vi "FilePath.vi"() -> (3 "添加的路径":path)   [LabVIEW 2018]
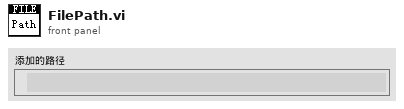
[diagram p1: front panel]
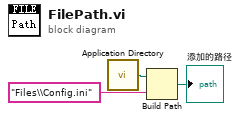
[diagram p0: block diagram]
diagram:
  n1 = call <vilib>:"Application Directory.vi"() -> ("Application Directory"=w3:path)
  n2 = Build Path(base path=w3, name or relative path="Files\\Config.ini" ("名称或相对路径")) -> (appended path=→"添加的路径":path)
